vi "DataVIS_Read Index .DAT Data.vi"(8 "error in (no error)":errorcluster, 11 "file path (use dialog)":path) -> (0 "error out":errorcluster, 2 "itx # info":i32[](array[numeric]), 3 "channel / path dictionary":T1)   [LabVIEW 2016]
uses:
  <userlib>/_OpenG.lib/dictionary/dictionary.llb/Dictionary Object RefNum__ogtk.ctl
  <userlib>/_OpenG.lib/dictionary/dictionary.llb/Dictionary Object RefNum - Enum__ogtk.ctl
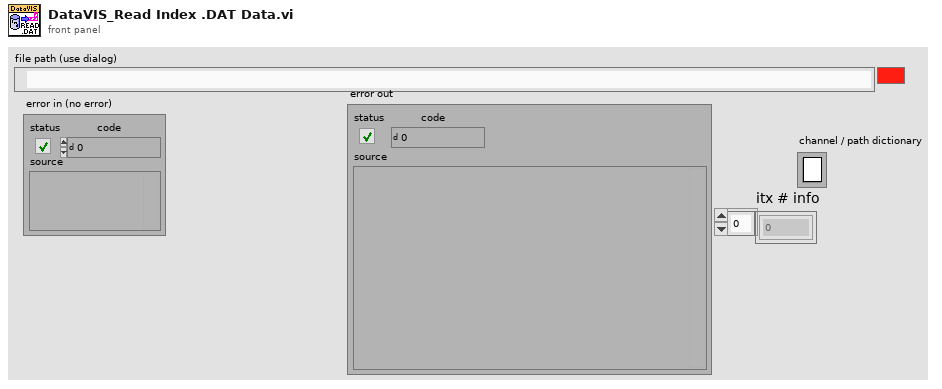
[diagram p1: front panel]
types:
  T1 = typedef "Dictionary Object RefNum__ogtk.ctl" = refnum<k1>
  T2 = cluster{"items":cluster{string, path}[], "itx # info":i32[]}
  T3 = enum16{"open", "replace", "create", "open or create", "replace or create", "replace or create with confirmation"}
  T4 = cluster{"items":cluster{string, path}[], "itx # info":i32[]}[]
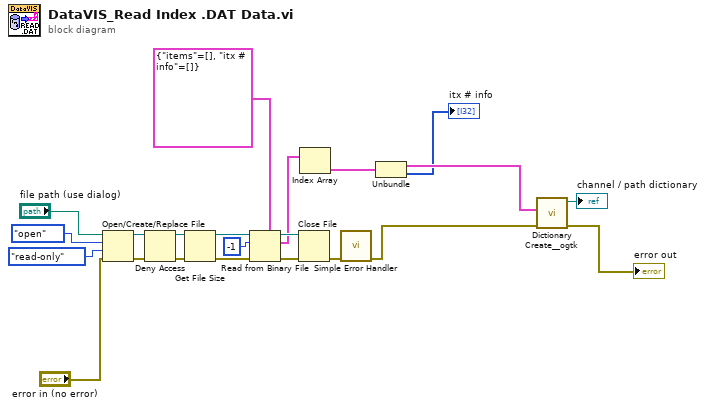
[diagram p0: block diagram]
diagram:
  n1 = Open/Create/Replace File(file path (use dialog)="file path (use dialog)", error in="error in (no error)", operation (0:open)=T3."open", access (0:read/write)=enum16{"read/write", "read-only", "write-only"}."read-only") -> (refnum out=w17:refnum<file>, error out=w16:errorcluster)  [unwired: 2 in, 1 out]
  n2 = Deny Access(4:w16, 7:w17) -> (0:w18:errorcluster, 3:w19:refnum<file>)  [unwired: 1 in]
  n3 = Get File Size(file=w19, error in=w18) -> (refnum out=w10:refnum<file>, 0:w14:errorcluster)  [unwired: 1 out]
  n4 = Read from Binary File(5:T2 {"items"=[], "itx # info"=[]}, 8:w14, 10:-1 ("count (1)"), 11:w10) -> (0:w12:errorcluster, 2:w4:T4, 3:w11:refnum<file>)  [unwired: 2 in, 1 out]
  n5 = Close File(refnum=w11, error in=w12) -> (error out=w13:errorcluster)  [unwired: 1 out]
  n6 = Index Array(array=w4) -> (element=w3:T2)  [unwired: 1 in]
  n7 = call <vilib>:"Simple Error Handler.vi"("error in (no error)"=w13) -> ("error out"=w8:errorcluster)  [unwired: 4 in, 4 out]
  n8 = Unbundle(w3) -> ("items"=w2:cluster{string, path}[], "itx # info"=→"itx # info":i32[])
  n9 = call <userlib>:"Dictionary Create__ogtk.vi"("error in (no error)"=w8, "initial dictionary (empty)"=w2) -> ("error out"=→"error out":errorcluster, "dictionary out"=→"channel / path dictionary":T1)  [unwired: 8 in]
